vi "Write Delimited Spreadsheet String.vi"(7 "prompt":string, 8 "error in":errorcluster, 9 "append to file?":bool, 10 "spreadsheet string":string, 11 "Path":path) -> (0 "error out":errorcluster, 3 "path":path)   [LabVIEW 2018]
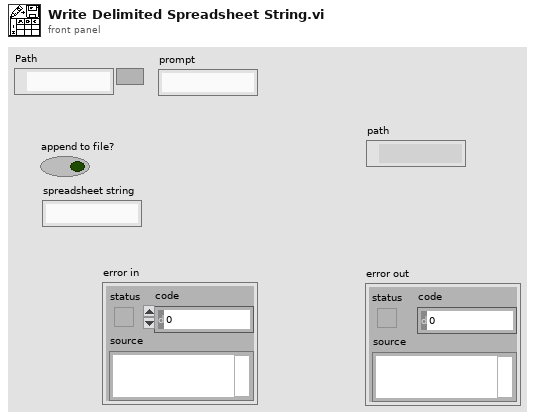
[diagram p1: front panel]
types:
  T1 = enum16{"open", "replace", "create", "open or create", "replace or create", "replace or create with confirmation"}
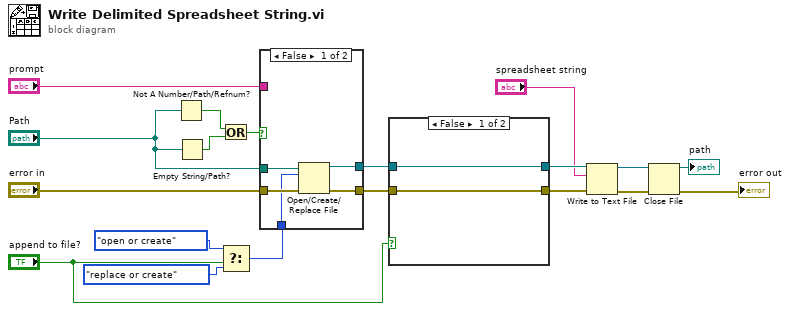
[diagram p0: block diagram]
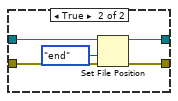
[diagram p2: hidden frame]
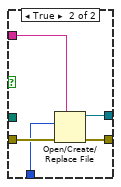
[diagram p3: hidden frame]
diagram:
  n1 = Not A Number/Path/Refnum?(number/path/refnum="Path") -> (NaN/Path/Refnum?=w19:bool)
  n2 = Empty String/Path?(string/path="Path") -> (empty?=w18:bool)
  n3 = Or(x=w19, y=w18) -> (x .or. y?=w17:bool)
  n4 = Select(t=T1."open or create" ("operation (0:open)"), s="append to file?", f=T1."replace or create" ("operation (0:open)")) -> (s? t:f=w11:T1)
  n5 = case shown="False" w17 {
    tunnel: "Path" -> [w23 _]
    tunnel: "prompt" -> [_ w29]
    tunnel: "error in" -> [w22 w28]
    tunnel: w11 -> [w21 w27]
    tunnel: [w20 w26] -> w9
    tunnel: [w24 w25] -> w8
    frame False {
      n6 = Open/Create/Replace File(file path (use dialog)=w23, error in=w22, operation (0:open)=w21) -> (refnum out=w20:refnum<file>, error out=w24:errorcluster)  [unwired: 3 in, 1 out]
    }
    frame True {
      n7 = Open/Create/Replace File(error in=w28, prompt=w29, operation (0:open)=w27) -> (refnum out=w26:refnum<file>, error out=w25:errorcluster)  [unwired: 3 in, 1 out]
    }
  }
  n8 = case shown="False" "append to file?" {
    tunnel: w9 -> [w31 w36]
    tunnel: w8 -> [w30 w35]
    tunnel: [w31 w33] -> w7
    tunnel: [w30 w32] -> w6
    frame False {
    }
    frame True {
      n9 = Set File Position(refnum=w36, from (0:start)=enum16{"start", "end", "current"}."end", error in=w35) -> (refnum out=w33:refnum<file>, error out=w32:errorcluster)  [unwired: 1 in]
    }
  }
  n10 = Write to Text File(file (use dialog)=w7, text="spreadsheet string", error in=w6) -> (refnum out=w3:refnum<file>, error out=w4:errorcluster)  [unwired: 1 in, 1 out]
  n11 = Close File(refnum=w3, error in=w4) -> (path=→"path":path, error out=→"error out":errorcluster)
